vi "Timer.vi"(8 "error in":errorcluster, 10 "Input Data":T2, 11 "Options":T3) -> (0 "error out":errorcluster, 3 "Output Data":T1)   [LabVIEW 2023, in "HardwareAbstractionLayer_LVOOP.lvlib" / "Wait Monitor.lvclass"]
uses:
  Wait Monitor.lvclass
  Control/TimerStates.ctl
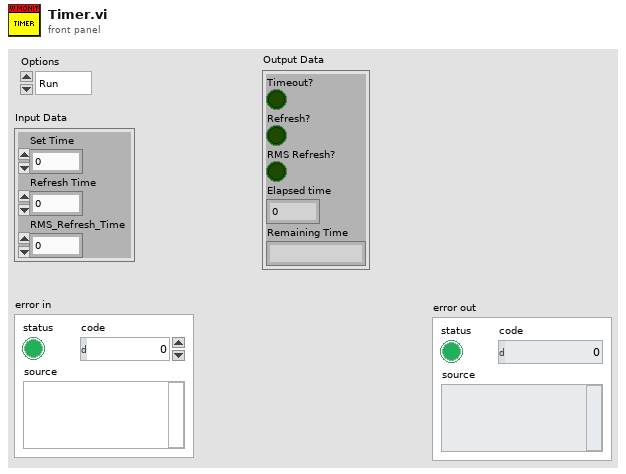
[diagram p1: front panel]
types:
  T1 = cluster{"Timeout?":bool, "Refresh?":bool, "RMS Refresh?":bool, "Elapsed time":dbl, "Remaining Time":string}
  T2 = cluster{"Set Time":dbl, "Refresh Time":dbl, "RMS_Refresh_Time":dbl}
  T3 = typedef "HardwareAbstractionLayer_LVOOP.lvlib/Wait Monitor.lvclass/TimerStates.ctl" = enum16{"Run", "Pause", "Reset"}
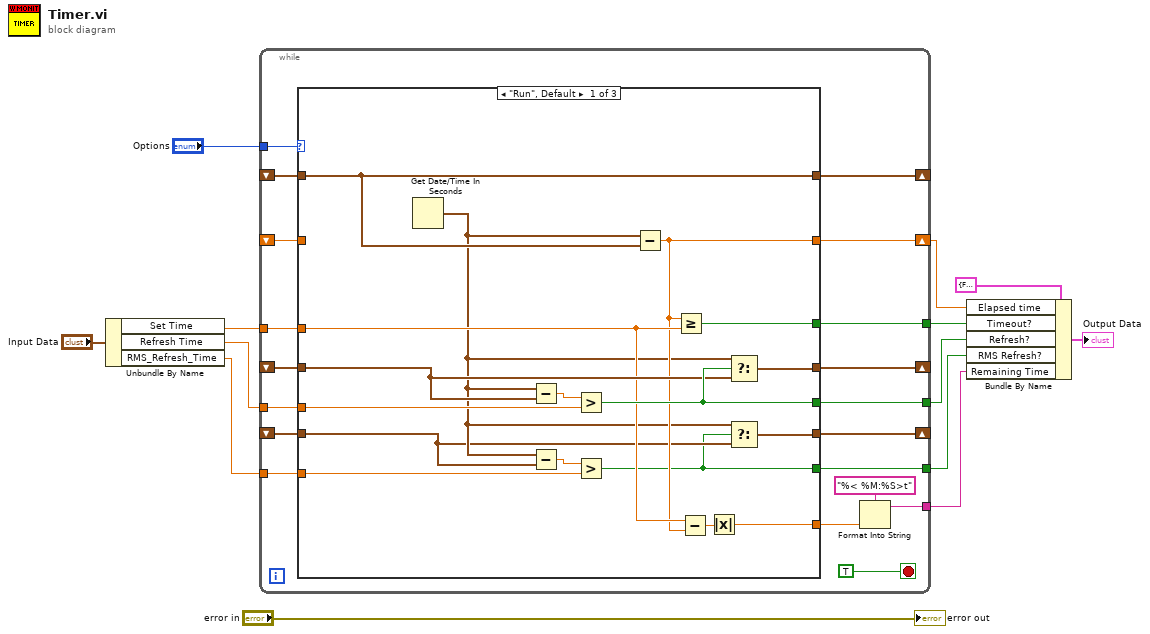
[diagram p0: block diagram]
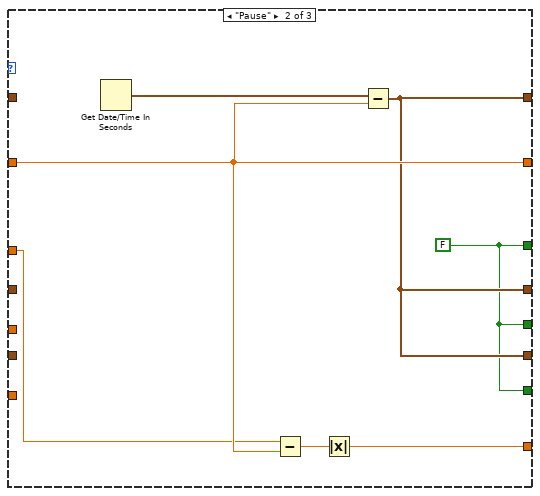
[diagram p2: hidden frame]
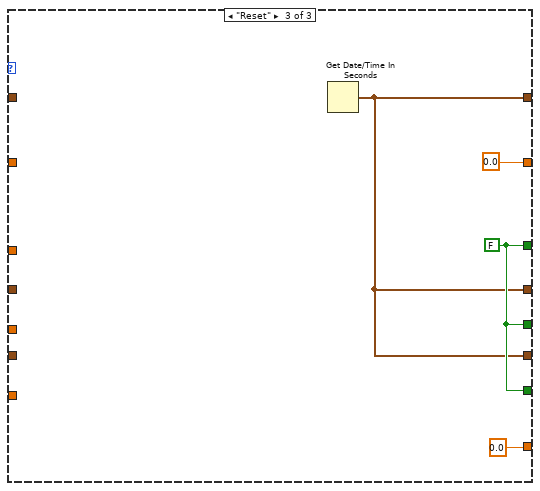
[diagram p3: hidden frame]
diagram:
  n1 = Unbundle By Name("Input Data") -> ("Set Time"=w10:dbl, "Refresh Time"=w9:dbl, "RMS_Refresh_Time"=w8:dbl)
  n2 = while {
    tunnel: "Options" -> [w32]
    shift-right: [w29] -> _
    shift-left: _ -> [w30]
    tunnel: w10 -> [w28]
    tunnel: [w26] -> w5
    shift-right: [w27] -> w6
    shift-left: _ -> [w25]
    tunnel: w9 -> [w24]
    tunnel: [w23] -> w4
    shift-right: [w22] -> _
    shift-left: _ -> [w21]
    tunnel: [w14] -> w1
    shift-right: [w20] -> _
    shift-left: _ -> [w19]
    tunnel: w8 -> [w18]
    tunnel: [w17] -> w3
    stop <- TRUE stop-if-true
    n3 = case shown="\"Run\", Default" w32 {
      tunnel: [w40 w55 0.0] -> w27
      tunnel: w30 -> [w49 _ _]
      tunnel: [w49 w52 w58] -> w29
      tunnel: [w48 w51 w59] -> w26
      tunnel: w28 -> [w41 w54 _]
      tunnel: w25 -> [_ w55 _]
      tunnel: w24 -> [w47 _ _]
      tunnel: [w46 w51 w59] -> w23
      tunnel: [w45 w52 w58] -> w22
      tunnel: w21 -> [w43 _ _]
      tunnel: [w37 w52 w58] -> w20
      tunnel: w19 -> [w35 _ _]
      tunnel: w18 -> [w36 _ _]
      tunnel: [w34 w51 w59] -> w17
      tunnel: [w33 w50 0.0] -> w15
      frame "Run", Default {
        n4 = Get Date/Time In Seconds() -> (seconds since 1Jan1904=w38:timestamp)
        n5 = Subtract(x=w38, y=w43) -> (x-y=w44:dbl)
        n6 = Subtract(x=w38, y=w35) -> (x-y=w39:dbl)
        n7 = Greater?(x=w44, y=w47) -> (0:w46:bool)
        n8 = Greater?(x=w39, y=w36) -> (0:w34:bool)
        n9 = Subtract(x=w38, y=w49) -> (x-y=w40:dbl)
        n10 = Greater Or Equal?(x=w40, y=w41) -> (x >= y?=w48:bool)
        n11 = Subtract(x=w41, y=w40) -> (x-y=w42:dbl)
        n12 = Absolute Value(x=w42) -> (abs(x)=w33:dbl)
        n13 = Select(t=w38, s=w46, f=w43) -> (s? t:f=w45:timestamp)
        n14 = Select(t=w38, s=w34, f=w35) -> (s? t:f=w37:timestamp)
      }
      frame "Pause" {
        w51 = FALSE
        n15 = Get Date/Time In Seconds() -> (seconds since 1Jan1904=w56:timestamp)
        n16 = Subtract(x=w54, y=w55) -> (x-y=w53:dbl)
        n17 = Absolute Value(x=w53) -> (abs(x)=w50:dbl)
        n18 = Subtract(x=w56, y=w55) -> (x-y=w52:timestamp)
      }
      frame "Reset" {
        w59 = FALSE
        n19 = Get Date/Time In Seconds() -> (seconds since 1Jan1904=w58:timestamp)
      }
    }
    n20 = Format Into String(format string="%< %M:%S>t", w15) -> (resulting string=w14:string)  [unwired: 2 in, 1 out]
  }
  n21 = Bundle By Name(cluster=T1 {"Timeout?"=FALSE, "Refresh?"=FALSE, "RMS Refresh?"=FALSE, "Elapsed time"=0.0, "Remaining Time"=""} ("Output Data"), "Elapsed time"=w6, "Timeout?"=w5, "Refresh?"=w4, "RMS Refresh?"=w3, "Remaining Time"=w1) -> (→"Output Data":T1)
  "error out" <- "error in"
